vi "Channel_Manager2.vi"() -> ()   [LabVIEW 2018]
uses:
  CCDCamera/CCDCamera.lvclass
  RxTx/RxTx.lvclass
  Cooler/Cooler.lvclass
  Interface/Interface.lvclass
  Channel Manager/Channel Manager.lvclass
  Readout delay charact/Readout Delay Charact/Readout Charact.lvclass
  Save Images/Save Images.lvclass
  Product/Product.lvclass
  Creator/Creator.lvclass
panel:
  in  "Channel Manager in":refnum<class "Channel Manager.lvclass">
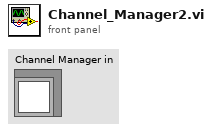
[diagram p1: front panel]
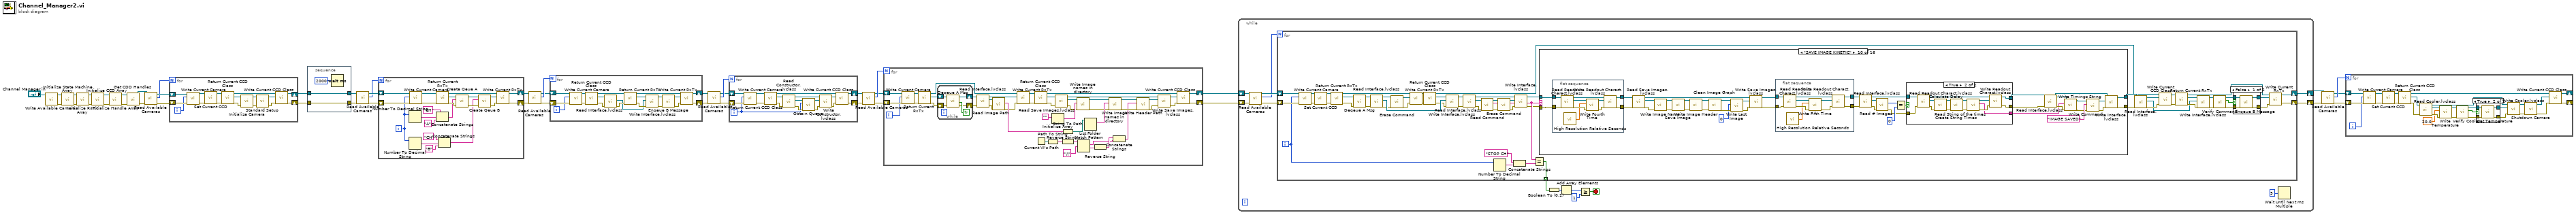
[diagram p0: block diagram]
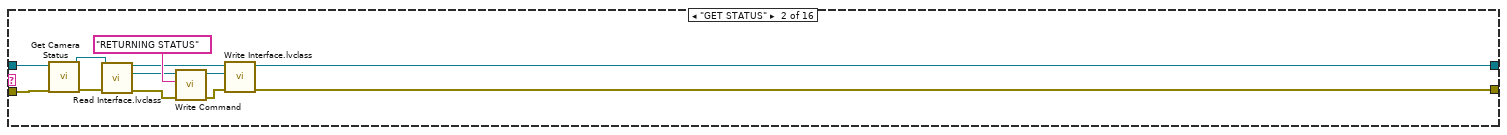
[diagram p4: hidden frame]
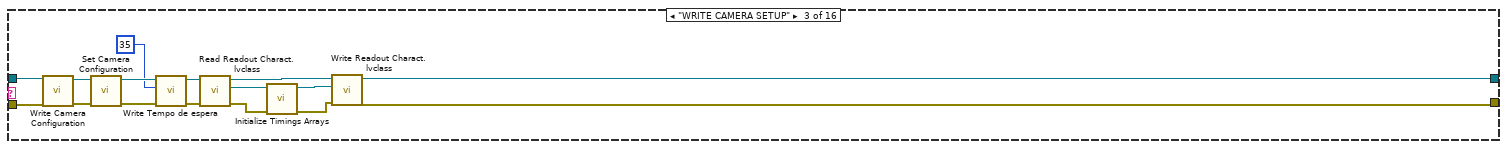
[diagram p5: hidden frame]
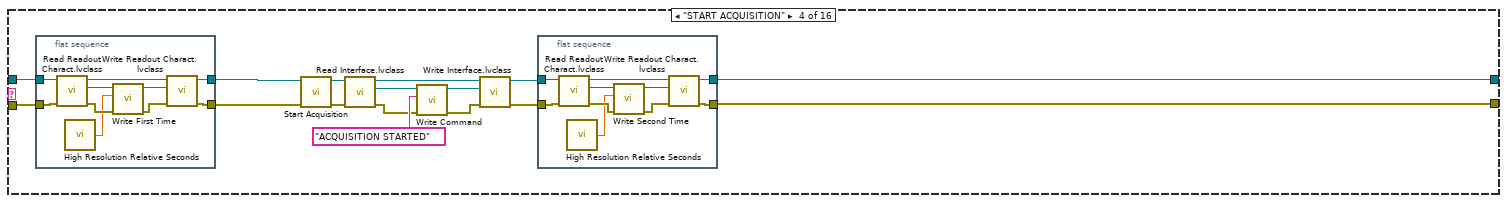
[diagram p6: hidden frame]
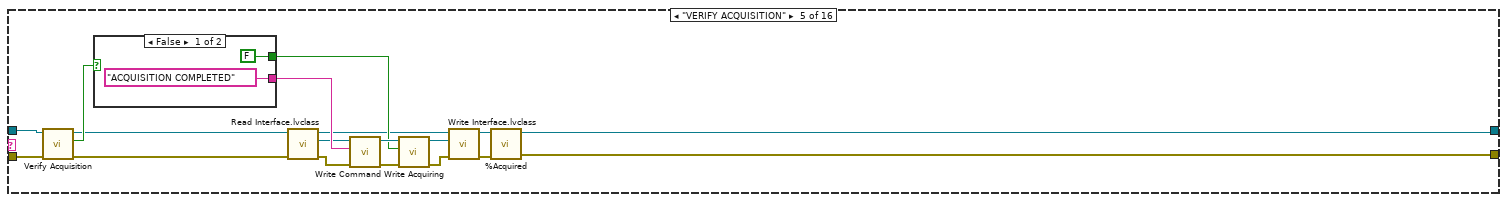
[diagram p7: hidden frame]
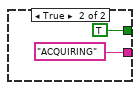
[diagram p8: hidden frame]
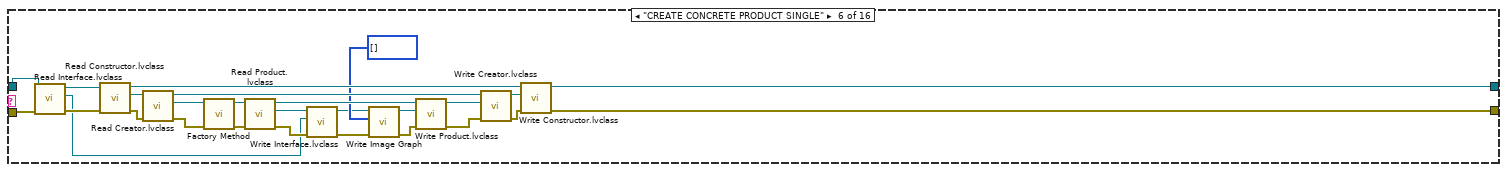
[diagram p9: hidden frame]
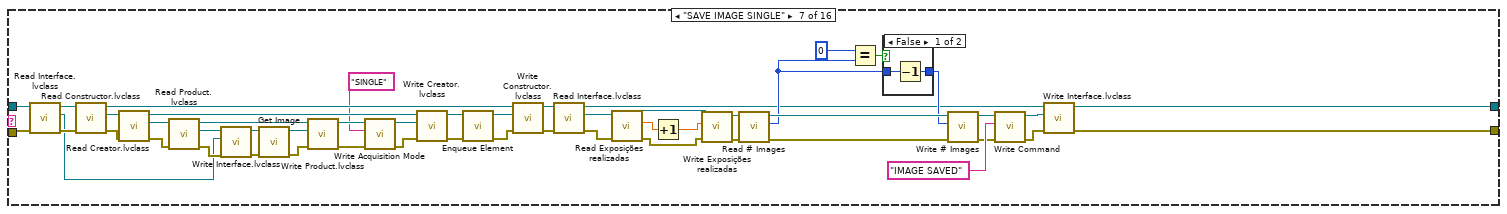
[diagram p10: hidden frame]
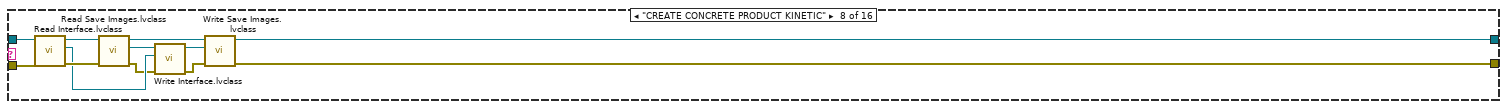
[diagram p12: hidden frame]
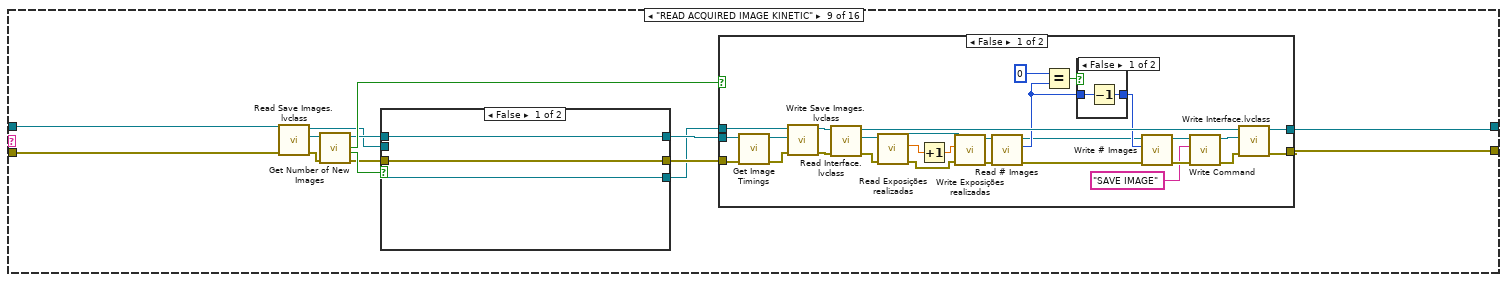
[diagram p13: hidden frame]
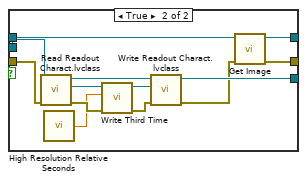
[diagram p14: hidden frame]
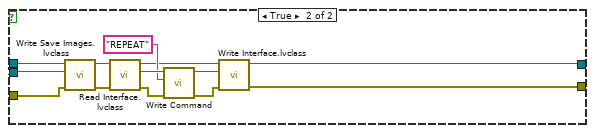
[diagram p16: hidden frame]
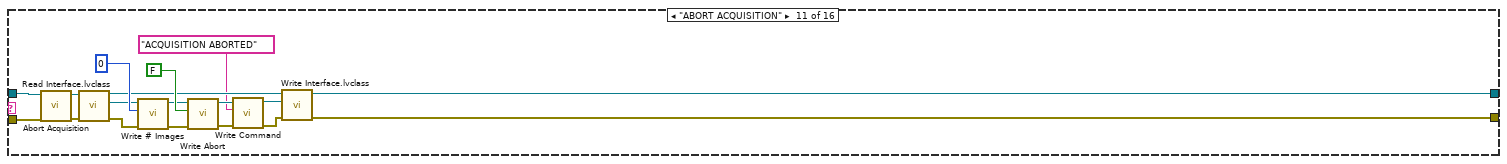
[diagram p18: hidden frame]
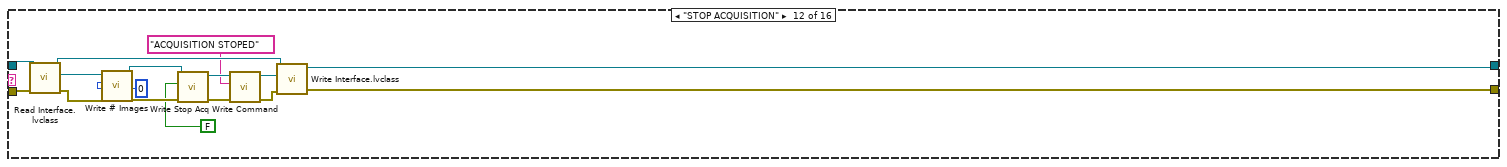
[diagram p19: hidden frame]
diagram:
  n1 = call-dynamic "Write Available Cameras.vi"("Channel Manager in"="Channel Manager in") -> ("error out"=w28:errorcluster, "Channel Manager out"=w27:refnum<class "Channel Manager.lvclass">)  [unwired: 9 in]
  n2 = call "Initialize State Machine Array.vi"("error in (no error)"=w28, "Channel Manager in"=w27) -> ("error out"=w36:errorcluster, "Channel Manager out"=w41:refnum<class "Channel Manager.lvclass">)  [unwired: 8 in]
  n3 = call "Initialize RxTx Array.vi"("error in (no error)"=w36, "Channel Manager in"=w41) -> ("error out"=w37:errorcluster, "Channel Manager out"=w40:refnum<class "Channel Manager.lvclass">)  [unwired: 8 in]
  n4 = call "Initialize CCD Array.vi"("error in (no error)"=w37, "Channel Manager in"=w40) -> ("error out"=w38:errorcluster, "Channel Manager out"=w39:refnum<class "Channel Manager.lvclass">)  [unwired: 8 in]
  n5 = call "Initialize Handle Array.vi"("error in (no error)"=w38, "Channel Manager in"=w39) -> ("error out"=w35:errorcluster, "Channel Manager out"=w34:refnum<class "Channel Manager.lvclass">)  [unwired: 8 in]
  n6 = call "Get CDD Handles.vi"("error in (no error)"=w35, "Channel Manager in"=w34) -> ("error out"=w33:errorcluster, "Channel Manager out"=w32:refnum<class "Channel Manager.lvclass">)  [unwired: 8 in]
  n7 = call-dynamic "Read Available Cameras.vi"("error in (no error)"=w33, "Channel Manager in"=w32) -> ("error out"=w30:errorcluster, "Available Cameras"=w29:u8, "Channel Manager out"=w31:refnum<class "Channel Manager.lvclass">)  [unwired: 7 in]
  n8 = for {
    N: w29 -> [_]
    shift-right: [w52] -> w45
    shift-left: w31 -> [w48]
    shift-right: [w51] -> w44
    shift-left: w30 -> [w47]
    i -> [w46]
    n9 = call-dynamic "Write Current Camera.vi"("error in (no error)"=w47, "Current Camera"=w46, "Channel Manager in"=w48) -> ("error out"=w50:errorcluster, "Channel Manager out"=w49:refnum<class "Channel Manager.lvclass">)  [unwired: 7 in]
    n10 = call "Set Current CCD.vi"("error in (no error)"=w50, "Channel Manager in"=w49) -> ("error out"=w55:errorcluster, "Channel Manager out"=w56:refnum<class "Channel Manager.lvclass">)  [unwired: 8 in]
    n11 = call "Return Current CCD Class.vi"("error in (no error)"=w55, "Channel Manager in"=w56) -> ("error out"=w60:errorcluster, "CCD Class"=w61:refnum<class "CCDCamera.lvclass">, "Channel Manager out"=w59:refnum<class "Channel Manager.lvclass">)  [unwired: 7 in]
    n12 = call "Initialize Camera.vi"("error in (no error)"=w60, "CCDCamera in"=w61) -> ("error out"=w58:errorcluster, "CCDCamera out"=w57:refnum<class "CCDCamera.lvclass">)  [unwired: 8 in]
    n13 = call "Standard Setup.vi"("error in (no error)"=w58, "CCDCamera in"=w57) -> ("error out"=w54:errorcluster, "CCDCamera out"=w53:refnum<class "CCDCamera.lvclass">)  [unwired: 8 in]
    n14 = call "Write Current CCD Class.vi"("error in (no error)"=w54, "CCD Class"=w53, "Channel Manager in"=w59) -> ("error out"=w51:errorcluster, "Channel Manager out"=w52:refnum<class "Channel Manager.lvclass">)  [unwired: 7 in]
  }
  n15 = stacked-sequence {
    tunnel: w45 -> [w63]
    tunnel: w44 -> [w62]
    tunnel: [w63] -> w24
    tunnel: [w62] -> w25
    frame #0 {
      n16 = Wait (ms)(milliseconds to wait=u32 2000) -> ()  [unwired: 1 out]
    }
  }
  n17 = call-dynamic "Read Available Cameras.vi"("error in (no error)"=w25, "Channel Manager in"=w24) -> ("error out"=w22:errorcluster, "Available Cameras"=w21:u8, "Channel Manager out"=w23:refnum<class "Channel Manager.lvclass">)  [unwired: 7 in]
  n18 = for {
    N: w21 -> [_]
    shift-right: [w71] -> w19
    shift-left: w23 -> [w66]
    shift-right: [w70] -> w20
    shift-left: w22 -> [w67]
    i -> [w65]
    n19 = Number To Decimal String(number=w65) -> (decimal integer string=w78:string)  [unwired: 1 in]
    n20 = Number To Decimal String(number=w65) -> (decimal integer string=w79:string)  [unwired: 1 in]
    n21 = call-dynamic "Write Current Camera.vi"("error in (no error)"=w67, "Current Camera"=w65, "Channel Manager in"=w66) -> ("error out"=w69:errorcluster, "Channel Manager out"=w68:refnum<class "Channel Manager.lvclass">)  [unwired: 7 in]
    n22 = call "Return Current RxTx.vi"("error in (no error)"=w69, "Channel Manager in"=w68) -> ("error out"=w86:errorcluster, "RxTx"=w76:refnum<class "RxTx.lvclass">, "Channel Manager out"=w83:refnum<class "Channel Manager.lvclass">)  [unwired: 7 in]
    n23 = Concatenate Strings("CH", w78, "A") -> (w80:string)
    n24 = Concatenate Strings("CH", w79, "B") -> (w81:string)
    n25 = call "Create Qeue A.vi"("error in (no error)"=w86, "Qeue A"=w80, "RxTx in"=w76) -> ("error out"=w84:errorcluster, "RxTx out"=w77:refnum<class "RxTx.lvclass">)  [unwired: 7 in]
    n26 = call "Create Qeue B.vi"("error in (no error)"=w84, "Qeue B"=w81, "RxTx in"=w77) -> ("error out"=w85:errorcluster, "RxTx out"=w82:refnum<class "RxTx.lvclass">)  [unwired: 7 in]
    n27 = call "Write Current RxTx.vi"("error in (no error)"=w85, "RxTx"=w82, "Channel Manager in"=w83) -> ("error out"=w70:errorcluster, "Channel Manager out"=w71:refnum<class "Channel Manager.lvclass">)  [unwired: 7 in]
  }
  n28 = call-dynamic "Read Available Cameras.vi"("error in (no error)"=w20, "Channel Manager in"=w19) -> ("error out"=w16:errorcluster, "Available Cameras"=w18:u8, "Channel Manager out"=w17:refnum<class "Channel Manager.lvclass">)  [unwired: 7 in]
  n29 = for {
    N: w18 -> [_]
    shift-right: [w93] -> w14
    shift-left: w17 -> [w89]
    shift-right: [w92] -> w15
    shift-left: w16 -> [w88]
    i -> [w87]
    n30 = call-dynamic "Write Current Camera.vi"("error in (no error)"=w88, "Current Camera"=w87, "Channel Manager in"=w89) -> ("error out"=w91:errorcluster, "Channel Manager out"=w90:refnum<class "Channel Manager.lvclass">)  [unwired: 7 in]
    n31 = call "Return Current CCD Class.vi"("error in (no error)"=w91, "Channel Manager in"=w90) -> ("error out"=w104:errorcluster, "CCD Class"=w105:refnum<class "CCDCamera.lvclass">, "Channel Manager out"=w102:refnum<class "Channel Manager.lvclass">)  [unwired: 7 in]
    n32 = call-dynamic "Read Interface.lvclass.vi"("error in (no error)"=w104, "CCDCamera in"=w105) -> ("error out"=w103:errorcluster, "Interface.lvclass"=w99:refnum<class "Interface.lvclass">)  [unwired: 7 in, 1 out]
    n33 = call "Return Current RxTx.vi"("error in (no error)"=w103, "Channel Manager in"=w102) -> ("error out"=w101:errorcluster, "RxTx"=w100:refnum<class "RxTx.lvclass">, "Channel Manager out"=w96:refnum<class "Channel Manager.lvclass">)  [unwired: 7 in]
    n34 = call-dynamic "Write Interface.lvclass.vi"("error in (no error)"=w101, "Interface.lvclass"=w99, "RxTx in"=w100) -> ("error out"=w98:errorcluster, "RxTx out"=w97:refnum<class "RxTx.lvclass">)  [unwired: 7 in]
    n35 = call "Enqeue B Message.vi"("error in (no error)"=w98, "RxTx in"=w97) -> ("error out"=w94:errorcluster, "RxTx out"=w95:refnum<class "RxTx.lvclass">)  [unwired: 8 in]
    n36 = call "Write Current RxTx.vi"("error in (no error)"=w94, "RxTx"=w95, "Channel Manager in"=w96) -> ("error out"=w92:errorcluster, "Channel Manager out"=w93:refnum<class "Channel Manager.lvclass">)  [unwired: 7 in]
  }
  n37 = call-dynamic "Read Available Cameras.vi"("error in (no error)"=w15, "Channel Manager in"=w14) -> ("error out"=w11:errorcluster, "Available Cameras"=w13:u8, "Channel Manager out"=w12:refnum<class "Channel Manager.lvclass">)  [unwired: 7 in]
  n38 = for {
    N: w13 -> [_]
    shift-right: [w112] -> w9
    shift-left: w12 -> [w108]
    shift-right: [w111] -> w10
    shift-left: w11 -> [w107]
    i -> [w106]
    n39 = call-dynamic "Write Current Camera.vi"("error in (no error)"=w107, "Current Camera"=w106, "Channel Manager in"=w108) -> ("error out"=w110:errorcluster, "Channel Manager out"=w109:refnum<class "Channel Manager.lvclass">)  [unwired: 7 in]
    n40 = call "Return Current CCD Class.vi"("error in (no error)"=w110, "Channel Manager in"=w109) -> ("error out"=w121:errorcluster, "CCD Class"=w122:refnum<class "CCDCamera.lvclass">, "Channel Manager out"=w113:refnum<class "Channel Manager.lvclass">)  [unwired: 7 in]
    n41 = call "Read Constructor.lvclass.vi"("error in (no error)"=w121, "CCDCamera in"=w122) -> ("error out"=w119:errorcluster, "Constructor.lvclass"=w120:refnum<class "Constructor.lvclass">, "CCDCamera out"=w116:refnum<class "CCDCamera.lvclass">)  [unwired: 7 in]
    n42 = call "Obtain Queue.vi"("error in (no error)"=w119, "Channel"=w106, "Constructor in"=w120) -> ("error out"=w118:errorcluster, "Constructor out"=w117:refnum<class "Constructor.lvclass">)  [unwired: 7 in]
    n43 = call "Write Constructor.lvclass.vi"("error in (no error)"=w118, "Constructor.lvclass"=w117, "CCDCamera in"=w116) -> ("error out"=w115:errorcluster, "CCDCamera out"=w114:refnum<class "CCDCamera.lvclass">)  [unwired: 7 in]
    n44 = call "Write Current CCD Class.vi"("error in (no error)"=w115, "CCD Class"=w114, "Channel Manager in"=w113) -> ("error out"=w111:errorcluster, "Channel Manager out"=w112:refnum<class "Channel Manager.lvclass">)  [unwired: 7 in]
  }
  n45 = call-dynamic "Read Available Cameras.vi"("error in (no error)"=w10, "Channel Manager in"=w9) -> ("error out"=w6:errorcluster, "Available Cameras"=w8:u8, "Channel Manager out"=w7:refnum<class "Channel Manager.lvclass">)  [unwired: 7 in]
  n46 = for {
    N: w8 -> [_]
    shift-right: [w159] -> w42
    shift-left: w7 -> [w154]
    shift-right: [w158] -> w43
    shift-left: w6 -> [w155]
    i -> [w153]
    n47 = call-dynamic "Write Current Camera.vi"("error in (no error)"=w155, "Current Camera"=w153, "Channel Manager in"=w154) -> ("error out"=w157:errorcluster, "Channel Manager out"=w156:refnum<class "Channel Manager.lvclass">)  [unwired: 7 in]
    n48 = call "Return Current RxTx.vi"("error in (no error)"=w157, "Channel Manager in"=w156) -> ("error out"=w167:errorcluster, "RxTx"=w166:refnum<class "RxTx.lvclass">, "Channel Manager out"=w162:refnum<class "Channel Manager.lvclass">)  [unwired: 7 in]
    n49 = while {
      shift-right: [w170] -> w164
      shift-left: w166 -> [w169]
      shift-right: [w171] -> w165
      shift-left: w167 -> [w168]
      stop <- w172 continue-if-true
      n50 = call "Deqeue A Msg.vi"("error in (no error)"=w168, "RxTx in"=w169) -> ("error out"=w171:errorcluster, "Timeout"=w172:bool, "RxTx out"=w170:refnum<class "RxTx.lvclass">)  [unwired: 7 in]
    }
    n51 = call-dynamic "Read Interface.lvclass.vi"("error in (no error)"=w165, "RxTx in"=w164) -> ("error out"=w141:errorcluster, "Interface.lvclass"=w142:refnum<class "Interface.lvclass">, "RxTx out"=w163:refnum<class "RxTx.lvclass">)  [unwired: 7 in]
    n52 = call-dynamic "Read Image Path.vi"("error in (no error)"=w141, "Interface in"=w142) -> ("error out"=w135:errorcluster, "Image Path"=w152:string)  [unwired: 7 in, 1 out]
    n53 = call "Write Current RxTx.vi"("error in (no error)"=w135, "RxTx"=w163, "Channel Manager in"=w162) -> ("error out"=w160:errorcluster, "Channel Manager out"=w161:refnum<class "Channel Manager.lvclass">)  [unwired: 7 in]
    n54 = call "Return Current CCD Class.vi"("error in (no error)"=w160, "Channel Manager in"=w161) -> ("error out"=w139:errorcluster, "CCD Class"=w140:refnum<class "CCDCamera.lvclass">, "Channel Manager out"=w136:refnum<class "Channel Manager.lvclass">)  [unwired: 7 in]
    n55 = Current VI's Path() -> (path=w130:path)
    n56 = Path To String(path=w130) -> (string=w129:string)
    n57 = Initialize Array("") -> (w147:string[])  [unwired: 1 in]
    n58 = call "Read Save Images.lvclass.vi"("error in (no error)"=w139, "CCDCamera in"=w140) -> ("error out"=w146:errorcluster, "Save Images.lvclass"=w145:refnum<class "Save Images.lvclass">, "CCDCamera out"=w144:refnum<class "CCDCamera.lvclass">)  [unwired: 7 in]
    n59 = Reverse String(1:w129) -> (0:w128:string)
    n60 = String To Path(string=w152) -> (path=w151:path)
    n61 = call "Write Image names in directory.vi"("error in (no error)"=w146, "Image names in directory"=w147, "Save Images in"=w145) -> ("error out"=w149:errorcluster, "Save Images out"=w148:refnum<class "Save Images.lvclass">)  [unwired: 7 in]
    n62 = Match Pattern(string=w128, regular expression="\\") -> (match substring=w124:string, after substring=w126:string)  [unwired: 1 in, 2 out]
    n63 = List Folder(path=w151) -> (filenames=w150:string[])  [unwired: 3 in, 3 out]
    n64 = Reverse String(1:w126) -> (0:w125:string)
    n65 = call "Write Image names in directory.vi"("error in (no error)"=w149, "Image names in directory"=w150, "Save Images in"=w148) -> ("error out"=w132:errorcluster, "Save Images out"=w133:refnum<class "Save Images.lvclass">)  [unwired: 7 in]
    n66 = Concatenate Strings(w125, w124) -> (w123:string)
    n67 = call-dynamic "Write Header Path.vi"("error in (no error)"=w132, "Header Path"=w123, "Save Images in"=w133) -> ("error out"=w131:errorcluster, "Save Images out"=w134:refnum<class "Save Images.lvclass">)  [unwired: 7 in]
    n68 = call "Write Save Images.lvclass.vi"("error in (no error)"=w131, "Save Images.lvclass"=w134, "CCDCamera in"=w144) -> ("error out"=w137:errorcluster, "CCDCamera out"=w138:refnum<class "CCDCamera.lvclass">)  [unwired: 7 in]
    n69 = call "Write Current CCD Class.vi"("error in (no error)"=w137, "CCD Class"=w138, "Channel Manager in"=w136) -> ("error out"=w158:errorcluster, "Channel Manager out"=w159:refnum<class "Channel Manager.lvclass">)  [unwired: 7 in]
  }
  n70 = while {
    shift-right: [w179] -> w4
    shift-left: w42 -> [w176]
    shift-right: [w178] -> w5
    shift-left: w43 -> [w177]
    stop <- w181 stop-if-true
    n71 = call-dynamic "Read Available Cameras.vi"("error in (no error)"=w177, "Channel Manager in"=w176) -> ("error out"=w174:errorcluster, "Available Cameras"=w173:u8, "Channel Manager out"=w175:refnum<class "Channel Manager.lvclass">)  [unwired: 7 in]
    n72 = for {
      N: w173 -> [_]
      tunnel: [w209] -> w185 mode=indexing
      shift-right: [w192] -> w179
      shift-left: w175 -> [w188]
      shift-right: [w191] -> w178
      shift-left: w174 -> [w187]
      i -> [w186]
      n73 = call-dynamic "Write Current Camera.vi"("error in (no error)"=w187, "Current Camera"=w186, "Channel Manager in"=w188) -> ("error out"=w190:errorcluster, "Channel Manager out"=w189:refnum<class "Channel Manager.lvclass">)  [unwired: 7 in]
      n74 = call "Set Current CCD.vi"("error in (no error)"=w190, "Channel Manager in"=w189) -> ("error out"=w235:errorcluster, "Channel Manager out"=w236:refnum<class "Channel Manager.lvclass">)  [unwired: 8 in]
      n75 = call "Return Current RxTx.vi"("error in (no error)"=w235, "Channel Manager in"=w236) -> ("error out"=w208:errorcluster, "RxTx"=w207:refnum<class "RxTx.lvclass">, "Channel Manager out"=w239:refnum<class "Channel Manager.lvclass">)  [unwired: 7 in]
      n76 = call "Deqeue A Msg.vi"("error in (no error)"=w208, "RxTx in"=w207) -> ("error out"=w198:errorcluster, "RxTx out"=w197:refnum<class "RxTx.lvclass">)  [unwired: 7 in, 1 out]
      n77 = call-dynamic "Read Interface.lvclass.vi"("error in (no error)"=w198, "RxTx in"=w197) -> ("error out"=w196:errorcluster, "Interface.lvclass"=w241:refnum<class "Interface.lvclass">, "RxTx out"=w195:refnum<class "RxTx.lvclass">)  [unwired: 7 in]
      n78 = call "Erase Command.vi"("error in (no error)"=w196, "RxTx in"=w195) -> ("error out"=w193:errorcluster, "RxTx out"=w194:refnum<class "RxTx.lvclass">)  [unwired: 8 in]
      n79 = call "Write Current RxTx.vi"("error in (no error)"=w193, "RxTx"=w194, "Channel Manager in"=w239) -> ("error out"=w238:errorcluster, "Channel Manager out"=w237:refnum<class "Channel Manager.lvclass">)  [unwired: 7 in]
      n80 = call "Return Current CCD Class.vi"("error in (no error)"=w238, "Channel Manager in"=w237) -> ("error out"=w240:errorcluster, "CCD Class"=w242:refnum<class "CCDCamera.lvclass">, "Channel Manager out"=w222:refnum<class "Channel Manager.lvclass">)  [unwired: 7 in]
      n81 = call-dynamic "Write Interface.lvclass.vi"("error in (no error)"=w240, "Interface.lvclass"=w241, "CCDCamera in"=w242) -> ("error out"=w228:errorcluster, "CCDCamera out"=w229:refnum<class "CCDCamera.lvclass">)  [unwired: 7 in]
      n82 = call-dynamic "Read Interface.lvclass.vi"("error in (no error)"=w228, "CCDCamera in"=w229) -> ("error out"=w233:errorcluster, "Interface.lvclass"=w234:refnum<class "Interface.lvclass">, "CCDCamera out"=w206:refnum<class "CCDCamera.lvclass">)  [unwired: 7 in]
      n83 = call "Read Command.vi"("error in (no error)"=w233, "Interface in"=w234) -> ("error out"=w202:errorcluster, "Command"=w232:string, "Interface out"=w201:refnum<class "Interface.lvclass">)  [unwired: 7 in]
      n84 = Number To Decimal String(number=w186) -> (decimal integer string=w226:string)  [unwired: 1 in]
      n85 = call "Erase Command.vi"("error in (no error)"=w202, "Interface in"=w201) -> ("error out"=w199:errorcluster, "Interface out"=w200:refnum<class "Interface.lvclass">)  [unwired: 8 in]
      n86 = Concatenate Strings("STOP CH", w226) -> (w225:string)
      n87 = call-dynamic "Write Interface.lvclass.vi"("error in (no error)"=w199, "Interface.lvclass"=w200, "CCDCamera in"=w206) -> ("error out"=w204:errorcluster, "CCDCamera out"=w205:refnum<class "CCDCamera.lvclass">)  [unwired: 7 in]
      n88 = Equal?(x=w232, y=w225) -> (x = y?=w209:bool)
      n89 = case shown="\"SAVE IMAGE KINETIC\"" w232 {
        tunnel: w205 -> [w250 w262 w277 w285 w332 w347 w394 w428 w435 w525 w599 w612 w618 w630 w642 w655]
        tunnel: w204 -> [w249 w261 w278 w286 w331 w348 w395 w427 w434 w524 w600 w611 w617 w629 w641 w654]
        tunnel: [w250 w252 w264 w280 w318 w355 w410 w429 w431 w542 w588 w607 w618 w631 w639 w653] -> w230
        tunnel: [w249 w251 w263 w279 w317 w354 w409 w418 w430 w543 w589 w606 w617 w632 w640 w652] -> w231
        frame "False", Default {
        }
        frame "GET STATUS" {
          n90 = call "Get Camera Status.vi"("error in (no error)"=w261, "CCDCamera in"=w262) -> ("error out"=w260:errorcluster, "CCDCamera out"=w259:refnum<class "CCDCamera.lvclass">)  [unwired: 7 in, 1 out]
          n91 = call-dynamic "Read Interface.lvclass.vi"("error in (no error)"=w260, "CCDCamera in"=w259) -> ("error out"=w256:errorcluster, "Interface.lvclass"=w257:refnum<class "Interface.lvclass">, "CCDCamera out"=w253:refnum<class "CCDCamera.lvclass">)  [unwired: 7 in]
          n92 = call "Write Command.vi"("error in (no error)"=w256, "Command"="RETURNING STATUS", "Interface in"=w257) -> ("error out"=w255:errorcluster, "Interface out"=w254:refnum<class "Interface.lvclass">)  [unwired: 7 in]
          n93 = call-dynamic "Write Interface.lvclass.vi"("error in (no error)"=w255, "Interface.lvclass"=w254, "CCDCamera in"=w253) -> ("error out"=w251:errorcluster, "CCDCamera out"=w252:refnum<class "CCDCamera.lvclass">)  [unwired: 7 in]
        }
        frame "WRITE CAMERA SETUP" {
          n94 = call-dynamic "Write Camera Configuration.vi"("error in (no error)"=w278, "CCDCamera in"=w277) -> ("error out"=w276:errorcluster, "CCDCamera out"=w275:refnum<class "CCDCamera.lvclass">)  [unwired: 8 in]
          n95 = call "Set Camera Configuration.vi"("error in (no error)"=w276, "CCDCamera in"=w275) -> ("error out"=w274:errorcluster, "CCDCamera out"=w273:refnum<class "CCDCamera.lvclass">)  [unwired: 8 in]
          n96 = call-dynamic "Write Tempo de espera.vi"("error in (no error)"=w274, "Tempo de espera"=u16 35, "CCDCamera in"=w273) -> ("error out"=w271:errorcluster, "CCDCamera out"=w270:refnum<class "CCDCamera.lvclass">)  [unwired: 7 in]
          n97 = call-dynamic "Read Readout Charact.lvclass.vi"("error in (no error)"=w271, "CCDCamera in"=w270) -> ("error out"=w266:errorcluster, "Readout Charact.lvclass"=w269:refnum<class "Readout Charact.lvclass">, "CCDCamera out"=w265:refnum<class "CCDCamera.lvclass">)  [unwired: 7 in]
          n98 = call "Initialize Timings Arrays.vi"("error in (no error)"=w266, "Readout Charact in"=w269) -> ("error out"=w267:errorcluster, "Readout Charact out"=w268:refnum<class "Readout Charact.lvclass">)  [unwired: 8 in]
          n99 = call-dynamic "Write Readout Charact.lvclass.vi"("error in (no error)"=w267, "Readout Charact.lvclass"=w268, "CCDCamera in"=w265) -> ("error out"=w263:errorcluster, "CCDCamera out"=w264:refnum<class "CCDCamera.lvclass">)  [unwired: 7 in]
        }
        frame "START ACQUISITION" {
          n100 = flat-sequence {
            tunnel: w286 -> [w314]
            tunnel: w285 -> [w313]
            tunnel: [w312] -> w284
            tunnel: [w311] -> w283
            frame #0 {
              n101 = call-dynamic "Read Readout Charact.lvclass.vi"("error in (no error)"=w314, "CCDCamera in"=w313) -> ("error out"=w308:errorcluster, "Readout Charact.lvclass"=w309:refnum<class "Readout Charact.lvclass">, "CCDCamera out"=w305:refnum<class "CCDCamera.lvclass">)  [unwired: 7 in]
              n102 = call <vilib>:"High Resolution Relative Seconds.vi"() -> ("relative seconds"=w306:dbl)
              n103 = call-dynamic "Write First Time.vi"("error in (no error)"=w308, "First Time"=w306, "Readout Charact in"=w309) -> ("error out"=w307:errorcluster, "Readout Charact out"=w310:refnum<class "Readout Charact.lvclass">)  [unwired: 7 in]
              n104 = call-dynamic "Write Readout Charact.lvclass.vi"("error in (no error)"=w307, "Readout Charact.lvclass"=w310, "CCDCamera in"=w305) -> ("error out"=w311:errorcluster, "CCDCamera out"=w312:refnum<class "CCDCamera.lvclass">)  [unwired: 7 in]
            }
          }
          n105 = call "Start Acquisition.vi"("error in (no error)"=w283, "CCDCamera in"=w284) -> ("error out"=w292:errorcluster, "CCDCamera out"=w293:refnum<class "CCDCamera.lvclass">)  [unwired: 8 in]
          n106 = call-dynamic "Read Interface.lvclass.vi"("error in (no error)"=w292, "CCDCamera in"=w293) -> ("error out"=w287:errorcluster, "Interface.lvclass"=w291:refnum<class "Interface.lvclass">, "CCDCamera out"=w289:refnum<class "CCDCamera.lvclass">)  [unwired: 7 in]
          n107 = call "Write Command.vi"("error in (no error)"=w287, "Command"="ACQUISITION STARTED", "Interface in"=w291) -> ("error out"=w288:errorcluster, "Interface out"=w290:refnum<class "Interface.lvclass">)  [unwired: 7 in]
          n108 = call-dynamic "Write Interface.lvclass.vi"("error in (no error)"=w288, "Interface.lvclass"=w290, "CCDCamera in"=w289) -> ("error out"=w281:errorcluster, "CCDCamera out"=w282:refnum<class "CCDCamera.lvclass">)  [unwired: 7 in]
          n109 = flat-sequence {
            tunnel: w281 -> [w304]
            tunnel: w282 -> [w303]
            tunnel: [w302] -> w280
            tunnel: [w301] -> w279
            frame #0 {
              n110 = call-dynamic "Read Readout Charact.lvclass.vi"("error in (no error)"=w304, "CCDCamera in"=w303) -> ("error out"=w296:errorcluster, "Readout Charact.lvclass"=w297:refnum<class "Readout Charact.lvclass">, "CCDCamera out"=w300:refnum<class "CCDCamera.lvclass">)  [unwired: 7 in]
              n111 = call <vilib>:"High Resolution Relative Seconds.vi"() -> ("relative seconds"=w295:dbl)
              n112 = call-dynamic "Write Second Time.vi"("error in (no error)"=w296, "Second Time"=w295, "Readout Charact in"=w297) -> ("error out"=w299:errorcluster, "Readout Charact out"=w298:refnum<class "Readout Charact.lvclass">)  [unwired: 7 in]
              n113 = call-dynamic "Write Readout Charact.lvclass.vi"("error in (no error)"=w299, "Readout Charact.lvclass"=w298, "CCDCamera in"=w300) -> ("error out"=w301:errorcluster, "CCDCamera out"=w302:refnum<class "CCDCamera.lvclass">)  [unwired: 7 in]
            }
          }
        }
        frame "VERIFY ACQUISITION" {
          n114 = call "Verify Acquisition.vi"("error in (no error)"=w331, "CCDCamera in"=w332) -> ("error out"=w315:errorcluster, "Acquiring"=w330:bool, "CCDCamera out"=w316:refnum<class "CCDCamera.lvclass">)  [unwired: 7 in]
          n115 = case shown="False" w330 {
            tunnel: ["ACQUISITION COMPLETED" "ACQUIRING"] -> w329
            tunnel: [FALSE ("Acquiring") TRUE ("Acquiring")] -> w326
            frame False {
            }
            frame True {
            }
          }
          n116 = call-dynamic "Read Interface.lvclass.vi"("error in (no error)"=w315, "CCDCamera in"=w316) -> ("error out"=w324:errorcluster, "Interface.lvclass"=w325:refnum<class "Interface.lvclass">, "CCDCamera out"=w321:refnum<class "CCDCamera.lvclass">)  [unwired: 7 in]
          n117 = call "Write Command.vi"("error in (no error)"=w324, "Command"=w329, "Interface in"=w325) -> ("error out"=w328:errorcluster, "Interface out"=w327:refnum<class "Interface.lvclass">)  [unwired: 7 in]
          n118 = call-dynamic "Write Acquiring.vi"("error in (no error)"=w328, "Acquiring"=w326, "Interface in"=w327) -> ("error out"=w323:errorcluster, "Interface out"=w322:refnum<class "Interface.lvclass">)  [unwired: 7 in]
          n119 = call-dynamic "Write Interface.lvclass.vi"("error in (no error)"=w323, "Interface.lvclass"=w322, "CCDCamera in"=w321) -> ("error out"=w320:errorcluster, "CCDCamera out"=w319:refnum<class "CCDCamera.lvclass">)  [unwired: 7 in]
          n120 = call "%Acquired.vi"("error in (no error)"=w320, "CCDCamera in"=w319) -> ("error out"=w317:errorcluster, "CCDCamera out"=w318:refnum<class "CCDCamera.lvclass">)  [unwired: 8 in]
        }
        frame "CREATE CONCRETE PRODUCT SINGLE" {
          n121 = call-dynamic "Read Interface.lvclass.vi"("error in (no error)"=w348, "CCDCamera in"=w347) -> ("error out"=w345:errorcluster, "Interface.lvclass"=w342:refnum<class "Interface.lvclass">, "CCDCamera out"=w346:refnum<class "CCDCamera.lvclass">)  [unwired: 7 in]
          n122 = call "Read Constructor.lvclass.vi"("error in (no error)"=w345, "CCDCamera in"=w346) -> ("error out"=w358:errorcluster, "Constructor.lvclass"=w359:refnum<class "Constructor.lvclass">, "CCDCamera out"=w363:refnum<class "CCDCamera.lvclass">)  [unwired: 7 in]
          n123 = call "Read Creator.lvclass.vi"("error in (no error)"=w358, "Constructor in"=w359) -> ("error out"=w357:errorcluster, "Creator.lvclass"=w356:refnum<class "Creator.lvclass">, "Constructor out"=w362:refnum<class "Constructor.lvclass">)  [unwired: 7 in]
          n124 = call-dynamic "Factory Method.vi"("error in (no error)"=w357, "Creator in"=w356) -> ("error out"=w353:errorcluster, "Creator out"=w352:refnum<class "Creator.lvclass">)  [unwired: 8 in]
          n125 = call "Read Product.lvclass.vi"("error in (no error)"=w353, "Creator in"=w352) -> ("error out"=w344:errorcluster, "Product.lvclass"=w343:refnum<class "Product.lvclass">, "Creator out"=w351:refnum<class "Creator.lvclass">)  [unwired: 7 in]
          n126 = call "Write Interface.lvclass.vi"("error in (no error)"=w344, "Interface.lvclass"=w342, "Product in"=w343) -> ("error out"=w340:errorcluster, "Product out"=w339:refnum<class "Product.lvclass">)  [unwired: 7 in]
          n127 = call "Write Image Graph.vi"("error in (no error)"=w340, "Image Graph"=u16[] [], "Product in"=w339) -> ("error out"=w337:errorcluster, "Product out"=w338:refnum<class "Product.lvclass">)  [unwired: 7 in]
          n128 = call "Write Product.lvclass.vi"("error in (no error)"=w337, "Product.lvclass"=w338, "Creator in"=w351) -> ("error out"=w350:errorcluster, "Creator out"=w349:refnum<class "Creator.lvclass">)  [unwired: 7 in]
          n129 = call "Write Creator.lvclass.vi"("error in (no error)"=w350, "Creator.lvclass"=w349, "Constructor in"=w362) -> ("error out"=w361:errorcluster, "Constructor out"=w360:refnum<class "Constructor.lvclass">)  [unwired: 7 in]
          n130 = call "Write Constructor.lvclass.vi"("error in (no error)"=w361, "Constructor.lvclass"=w360, "CCDCamera in"=w363) -> ("error out"=w354:errorcluster, "CCDCamera out"=w355:refnum<class "CCDCamera.lvclass">)  [unwired: 7 in]
        }
        frame "SAVE IMAGE SINGLE" {
          n131 = call-dynamic "Read Interface.lvclass.vi"("error in (no error)"=w395, "CCDCamera in"=w394) -> ("error out"=w392:errorcluster, "Interface.lvclass"=w385:refnum<class "Interface.lvclass">, "CCDCamera out"=w393:refnum<class "CCDCamera.lvclass">)  [unwired: 7 in]
          n132 = call "Read Constructor.lvclass.vi"("error in (no error)"=w392, "CCDCamera in"=w393) -> ("error out"=w390:errorcluster, "Constructor.lvclass"=w391:refnum<class "Constructor.lvclass">, "CCDCamera out"=w378:refnum<class "CCDCamera.lvclass">)  [unwired: 7 in]
          n133 = call "Read Creator.lvclass.vi"("error in (no error)"=w390, "Constructor in"=w391) -> ("error out"=w388:errorcluster, "Creator.lvclass"=w389:refnum<class "Creator.lvclass">, "Constructor out"=w379:refnum<class "Constructor.lvclass">)  [unwired: 7 in]
          n134 = call "Read Product.lvclass.vi"("error in (no error)"=w388, "Creator in"=w389) -> ("error out"=w386:errorcluster, "Product.lvclass"=w387:refnum<class "Product.lvclass">, "Creator out"=w380:refnum<class "Creator.lvclass">)  [unwired: 7 in]
          n135 = call "Write Interface.lvclass.vi"("error in (no error)"=w386, "Interface.lvclass"=w385, "Product in"=w387) -> ("error out"=w383:errorcluster, "Product out"=w384:refnum<class "Product.lvclass">)  [unwired: 7 in]
          n136 = call-dynamic "Get Image.vi"("error in (no error)"=w383, "Product in"=w384) -> ("error out"=w382:errorcluster, "Product out"=w381:refnum<class "Product.lvclass">)  [unwired: 8 in]
          n137 = call "Write Product.lvclass.vi"("error in (no error)"=w382, "Product.lvclass"=w381, "Creator in"=w380) -> ("error out"=w365:errorcluster, "Creator out"=w366:refnum<class "Creator.lvclass">)  [unwired: 7 in]
          n138 = call "Write Acquisition Mode.vi"("error in (no error)"=w365, "Acquisition Mode"="SINGLE", "Creator in"=w366) -> ("error out"=w368:errorcluster, "Creator out"=w367:refnum<class "Creator.lvclass">)  [unwired: 7 in]
          n139 = call "Write Creator.lvclass.vi"("error in (no error)"=w368, "Creator.lvclass"=w367, "Constructor in"=w379) -> ("error out"=w372:errorcluster, "Constructor out"=w371:refnum<class "Constructor.lvclass">)  [unwired: 7 in]
          n140 = call "Enqueue Element.vi"("error in (no error)"=w372, "Constructor in"=w371) -> ("error out"=w369:errorcluster, "Constructor out"=w370:refnum<class "Constructor.lvclass">)  [unwired: 8 in]
          n141 = call "Write Constructor.lvclass.vi"("error in (no error)"=w369, "Constructor.lvclass"=w370, "CCDCamera in"=w378) -> ("error out"=w377:errorcluster, "CCDCamera out"=w376:refnum<class "CCDCamera.lvclass">)  [unwired: 7 in]
          n142 = call-dynamic "Read Interface.lvclass.vi"("error in (no error)"=w377, "CCDCamera in"=w376) -> ("error out"=w374:errorcluster, "Interface.lvclass"=w375:refnum<class "Interface.lvclass">, "CCDCamera out"=w373:refnum<class "CCDCamera.lvclass">)  [unwired: 7 in]
          n143 = call-dynamic "Read Exposições realizadas.vi"("error in (no error)"=w374, "Interface in"=w375) -> ("error out"=w411:errorcluster, "Exposições realizadas"=w414:dbl, "Interface out"=w412:refnum<class "Interface.lvclass">)  [unwired: 7 in]
          n144 = Increment(x=w414) -> (x+1=w413:dbl)
          n145 = call-dynamic "Write Exposições realizadas.vi"("error in (no error)"=w411, "Exposições realizadas"=w413, "Interface in"=w412) -> ("error out"=w405:errorcluster, "Interface out"=w404:refnum<class "Interface.lvclass">)  [unwired: 7 in]
          n146 = call-dynamic "Read # Images.vi"("error in (no error)"=w405, "Interface in"=w404) -> ("error out"=w402:errorcluster, "# Images"=w396:u32, "Interface out"=w403:refnum<class "Interface.lvclass">)  [unwired: 7 in]
          n147 = Equal?(x=u32 0, y=w396) -> (x = y?=w399:bool)
          n148 = case shown="False" w399 {
            tunnel: [w416 w417] -> w397
            tunnel: w396 -> [w415 w417]
            frame False {
              n149 = Decrement(x=w415) -> (x-1=w416:u32)
            }
            frame True {
            }
          }
          n150 = call-dynamic "Write # Images.vi"("error in (no error)"=w402, "# Images"=w397, "Interface in"=w403) -> ("error out"=w401:errorcluster, "Interface out"=w400:refnum<class "Interface.lvclass">)  [unwired: 7 in]
          n151 = call "Write Command.vi"("error in (no error)"=w401, "Command"="IMAGE SAVED", "Interface in"=w400) -> ("error out"=w408:errorcluster, "Interface out"=w407:refnum<class "Interface.lvclass">)  [unwired: 7 in]
          n152 = call-dynamic "Write Interface.lvclass.vi"("error in (no error)"=w408, "Interface.lvclass"=w407, "CCDCamera in"=w373) -> ("error out"=w409:errorcluster, "CCDCamera out"=w410:refnum<class "CCDCamera.lvclass">)  [unwired: 7 in]
        }
        frame "CREATE CONCRETE PRODUCT KINETIC" {
          n153 = call-dynamic "Read Interface.lvclass.vi"("error in (no error)"=w427, "CCDCamera in"=w428) -> ("error out"=w425:errorcluster, "Interface.lvclass"=w424:refnum<class "Interface.lvclass">, "CCDCamera out"=w426:refnum<class "CCDCamera.lvclass">)  [unwired: 7 in]
          n154 = call "Read Save Images.lvclass.vi"("error in (no error)"=w425, "CCDCamera in"=w426) -> ("error out"=w422:errorcluster, "Save Images.lvclass"=w423:refnum<class "Save Images.lvclass">, "CCDCamera out"=w419:refnum<class "CCDCamera.lvclass">)  [unwired: 7 in]
          n155 = call-dynamic "Write Interface.lvclass.vi"("error in (no error)"=w422, "Interface.lvclass"=w424, "Save Images in"=w423) -> ("error out"=w421:errorcluster, "Save Images out"=w420:refnum<class "Save Images.lvclass">)  [unwired: 7 in]
          n156 = call "Write Save Images.lvclass.vi"("error in (no error)"=w421, "Save Images.lvclass"=w420, "CCDCamera in"=w419) -> ("error out"=w418:errorcluster, "CCDCamera out"=w429:refnum<class "CCDCamera.lvclass">)  [unwired: 7 in]
        }
        frame "READ ACQUIRED IMAGE KINETIC" {
          n157 = call "Read Save Images.lvclass.vi"("error in (no error)"=w434, "CCDCamera in"=w435) -> ("error out"=w440:errorcluster, "Save Images.lvclass"=w438:refnum<class "Save Images.lvclass">, "CCDCamera out"=w433:refnum<class "CCDCamera.lvclass">)  [unwired: 7 in]
          n158 = call-dynamic "Get Number of New Images.vi"("error in (no error)"=w440, "Save Images in"=w438) -> ("error out"=w441:errorcluster, "Are the any new img ?"=w443:bool, "Are there any remaining img?"=w442:bool, "Save Images out"=w439:refnum<class "Save Images.lvclass">)  [unwired: 6 in]
          n159 = case shown="False" w443 {
            tunnel: w439 -> [w446 w459]
            tunnel: w441 -> [w445 w450]
            tunnel: [w446 w458] -> w436
            tunnel: [w445 w457] -> w437
            tunnel: w433 -> [w444 w449]
            tunnel: [w444 w448] -> w432
            frame False {
            }
            frame True {
              n160 = call-dynamic "Read Readout Charact.lvclass.vi"("error in (no error)"=w450, "CCDCamera in"=w449) -> ("error out"=w452:errorcluster, "Readout Charact.lvclass"=w455:refnum<class "Readout Charact.lvclass">, "CCDCamera out"=w456:refnum<class "CCDCamera.lvclass">)  [unwired: 7 in]
              n161 = call <vilib>:"High Resolution Relative Seconds.vi"() -> ("relative seconds"=w451:dbl)
              n162 = call-dynamic "Write Third Time.vi"("error in (no error)"=w452, "Third Time"=w451, "Readout Charact in"=w455) -> ("error out"=w453:errorcluster, "Readout Charact out"=w454:refnum<class "Readout Charact.lvclass">)  [unwired: 7 in]
              n163 = call-dynamic "Write Readout Charact.lvclass.vi"("error in (no error)"=w453, "Readout Charact.lvclass"=w454, "CCDCamera in"=w456) -> ("error out"=w447:errorcluster, "CCDCamera out"=w448:refnum<class "CCDCamera.lvclass">)  [unwired: 7 in]
              n164 = call-dynamic "Get Image.vi"("error in (no error)"=w447, "Save Images in"=w459) -> ("error out"=w457:errorcluster, "Save Images out"=w458:refnum<class "Save Images.lvclass">)  [unwired: 8 in]
            }
          }
          n165 = case shown="False" w442 {
            tunnel: w432 -> [w464 w496]
            tunnel: [w468 w497] -> w430
            tunnel: [w467 w498] -> w431
            tunnel: w436 -> [w463 w495]
            tunnel: w437 -> [w462 w494]
            frame False {
              n166 = call-dynamic "Get Image Timings.vi"("error in (no error)"=w462, "Save Images in"=w463) -> ("error out"=w460:errorcluster, "Save Images out"=w461:refnum<class "Save Images.lvclass">)  [unwired: 8 in]
              n167 = call "Write Save Images.lvclass.vi"("error in (no error)"=w460, "Save Images.lvclass"=w461, "CCDCamera in"=w464) -> ("error out"=w466:errorcluster, "CCDCamera out"=w465:refnum<class "CCDCamera.lvclass">)  [unwired: 7 in]
              n168 = call-dynamic "Read Interface.lvclass.vi"("error in (no error)"=w466, "CCDCamera in"=w465) -> ("error out"=w476:errorcluster, "Interface.lvclass"=w475:refnum<class "Interface.lvclass">, "CCDCamera out"=w488:refnum<class "CCDCamera.lvclass">)  [unwired: 7 in]
              n169 = call-dynamic "Read Exposições realizadas.vi"("error in (no error)"=w476, "Interface in"=w475) -> ("error out"=w474:errorcluster, "Exposições realizadas"=w471:dbl, "Interface out"=w473:refnum<class "Interface.lvclass">)  [unwired: 7 in]
              n170 = Increment(x=w471) -> (x+1=w472:dbl)
              n171 = call-dynamic "Write Exposições realizadas.vi"("error in (no error)"=w474, "Exposições realizadas"=w472, "Interface in"=w473) -> ("error out"=w477:errorcluster, "Interface out"=w478:refnum<class "Interface.lvclass">)  [unwired: 7 in]
              n172 = call-dynamic "Read # Images.vi"("error in (no error)"=w477, "Interface in"=w478) -> ("error out"=w480:errorcluster, "# Images"=w483:u32, "Interface out"=w479:refnum<class "Interface.lvclass">)  [unwired: 7 in]
              n173 = Equal?(x=u32 0, y=w483) -> (x = y?=w481:bool)
              n174 = case shown="False" w481 {
                tunnel: [w490 w491] -> w482
                tunnel: w483 -> [w489 w491]
                frame False {
                  n175 = Decrement(x=w489) -> (x-1=w490:u32)
                }
                frame True {
                }
              }
              n176 = call-dynamic "Write # Images.vi"("error in (no error)"=w480, "# Images"=w482, "Interface in"=w479) -> ("error out"=w484:errorcluster, "Interface out"=w485:refnum<class "Interface.lvclass">)  [unwired: 7 in]
              n177 = call "Write Command.vi"("error in (no error)"=w484, "Command"="SAVE IMAGE", "Interface in"=w485) -> ("error out"=w486:errorcluster, "Interface out"=w487:refnum<class "Interface.lvclass">)  [unwired: 7 in]
              n178 = call-dynamic "Write Interface.lvclass.vi"("error in (no error)"=w486, "Interface.lvclass"=w487, "CCDCamera in"=w488) -> ("error out"=w468:errorcluster, "CCDCamera out"=w467:refnum<class "CCDCamera.lvclass">)  [unwired: 7 in]
            }
            frame True {
              n179 = call "Write Save Images.lvclass.vi"("error in (no error)"=w494, "Save Images.lvclass"=w495, "CCDCamera in"=w496) -> ("error out"=w492:errorcluster, "CCDCamera out"=w493:refnum<class "CCDCamera.lvclass">)  [unwired: 7 in]
              n180 = call-dynamic "Read Interface.lvclass.vi"("error in (no error)"=w492, "CCDCamera in"=w493) -> ("error out"=w504:errorcluster, "Interface.lvclass"=w503:refnum<class "Interface.lvclass">, "CCDCamera out"=w501:refnum<class "CCDCamera.lvclass">)  [unwired: 7 in]
              n181 = call "Write Command.vi"("error in (no error)"=w504, "Command"="REPEAT", "Interface in"=w503) -> ("error out"=w499:errorcluster, "Interface out"=w500:refnum<class "Interface.lvclass">)  [unwired: 7 in]
              n182 = call-dynamic "Write Interface.lvclass.vi"("error in (no error)"=w499, "Interface.lvclass"=w500, "CCDCamera in"=w501) -> ("error out"=w497:errorcluster, "CCDCamera out"=w498:refnum<class "CCDCamera.lvclass">)  [unwired: 7 in]
            }
          }
        }
        frame "SAVE IMAGE KINETIC" {
          n183 = flat-sequence {
            tunnel: w524 -> [w582]
            tunnel: w525 -> [w581]
            tunnel: [w580] -> w527
            tunnel: [w579] -> w526
            frame #0 {
              n184 = call-dynamic "Read Readout Charact.lvclass.vi"("error in (no error)"=w582, "CCDCamera in"=w581) -> ("error out"=w574:errorcluster, "Readout Charact.lvclass"=w577:refnum<class "Readout Charact.lvclass">, "CCDCamera out"=w578:refnum<class "CCDCamera.lvclass">)  [unwired: 7 in]
              n185 = call <vilib>:"High Resolution Relative Seconds.vi"() -> ("relative seconds"=w573:dbl)
              n186 = call-dynamic "Write Fourth Time.vi"("error in (no error)"=w574, "Fourth Time"=w573, "Readout Charact in"=w577) -> ("error out"=w575:errorcluster, "Readout Charact out"=w576:refnum<class "Readout Charact.lvclass">)  [unwired: 7 in]
              n187 = call-dynamic "Write Readout Charact.lvclass.vi"("error in (no error)"=w575, "Readout Charact.lvclass"=w576, "CCDCamera in"=w578) -> ("error out"=w579:errorcluster, "CCDCamera out"=w580:refnum<class "CCDCamera.lvclass">)  [unwired: 7 in]
            }
          }
          n188 = call "Read Save Images.lvclass.vi"("error in (no error)"=w526, "CCDCamera in"=w527) -> ("error out"=w534:errorcluster, "Save Images.lvclass"=w535:refnum<class "Save Images.lvclass">, "CCDCamera out"=w533:refnum<class "CCDCamera.lvclass">)  [unwired: 7 in]
          n189 = call-dynamic "Write Image Name.vi"("error in (no error)"=w534, "Save Images in"=w535) -> ("error out"=w541:errorcluster, "Save Images out"=w539:refnum<class "Save Images.lvclass">)  [unwired: 7 in, 1 out]
          n190 = call-dynamic "Save Image.vi"("error in (no error)"=w541, "Save Images in"=w539) -> ("error out"=w540:errorcluster, "Save Images out"=w538:refnum<class "Save Images.lvclass">)  [unwired: 8 in]
          n191 = call-dynamic "Write Image Header.vi"("error in (no error)"=w540, "Save Images in"=w538) -> ("error out"=w537:errorcluster, "Save Images out"=w536:refnum<class "Save Images.lvclass">)  [unwired: 8 in]
          n192 = call-dynamic "Clean Image Graph.vi"("error in (no error)"=w537, "Save Images in"=w536) -> ("error out"=w532:errorcluster, "Save Images out"=w531:refnum<class "Save Images.lvclass">)  [unwired: 8 in]
          n193 = call "Write Last  Image.vi"("error in (no error)"=w532, "Last  Image"=0, "Save Images in"=w531) -> ("error out"=w528:errorcluster, "Save Images out"=w529:refnum<class "Save Images.lvclass">)  [unwired: 7 in]
          n194 = call "Write Save Images.lvclass.vi"("error in (no error)"=w528, "Save Images.lvclass"=w529, "CCDCamera in"=w533) -> ("error out"=w522:errorcluster, "CCDCamera out"=w523:refnum<class "CCDCamera.lvclass">)  [unwired: 7 in]
          n195 = flat-sequence {
            tunnel: w522 -> [w572]
            tunnel: w523 -> [w571]
            tunnel: [w564] -> w515
            tunnel: [w563] -> w516
            frame #0 {
              n196 = call-dynamic "Read Readout Charact.lvclass.vi"("error in (no error)"=w572, "CCDCamera in"=w571) -> ("error out"=w570:errorcluster, "Readout Charact.lvclass"=w569:refnum<class "Readout Charact.lvclass">, "CCDCamera out"=w565:refnum<class "CCDCamera.lvclass">)  [unwired: 7 in]
              n197 = call <vilib>:"High Resolution Relative Seconds.vi"() -> ("relative seconds"=w568:dbl)
              n198 = call-dynamic "Write Fifth Time.vi"("error in (no error)"=w570, "Fifth Time"=w568, "Readout Charact in"=w569) -> ("error out"=w566:errorcluster, "Readout Charact out"=w567:refnum<class "Readout Charact.lvclass">)  [unwired: 7 in]
              n199 = call-dynamic "Write Readout Charact.lvclass.vi"("error in (no error)"=w566, "Readout Charact.lvclass"=w567, "CCDCamera in"=w565) -> ("error out"=w563:errorcluster, "CCDCamera out"=w564:refnum<class "CCDCamera.lvclass">)  [unwired: 7 in]
            }
          }
          n200 = call-dynamic "Read Interface.lvclass.vi"("error in (no error)"=w516, "CCDCamera in"=w515) -> ("error out"=w513:errorcluster, "Interface.lvclass"=w514:refnum<class "Interface.lvclass">, "CCDCamera out"=w509:refnum<class "CCDCamera.lvclass">)  [unwired: 7 in]
          n201 = call-dynamic "Read # Images.vi"("error in (no error)"=w513, "Interface in"=w514) -> ("error out"=w508:errorcluster, "# Images"=w512:u32)  [unwired: 7 in, 1 out]
          n202 = Equal?(x=w512, y=0) -> (x = y?=w510:bool)
          n203 = case shown="True" w510 {
            tunnel: w509 -> [w548 w553]
            tunnel: w508 -> [w547 w552]
            tunnel: [w548 w551] -> w507
            tunnel: [w547 w550] -> w506
            tunnel: [_ w549] -> w505
            frame False {
            }
            frame True {
              n204 = call-dynamic "Read Readout Charact.lvclass.vi"("error in (no error)"=w552, "CCDCamera in"=w553) -> ("error out"=w560:errorcluster, "Readout Charact.lvclass"=w561:refnum<class "Readout Charact.lvclass">, "CCDCamera out"=w562:refnum<class "CCDCamera.lvclass">)  [unwired: 7 in]
              n205 = call "Calculate Delay.vi"("error in (no error)"=w560, "Readout Charact in"=w561) -> ("error out"=w554:errorcluster, "Readout Charact out"=w555:refnum<class "Readout Charact.lvclass">)  [unwired: 8 in]
              n206 = call "Create String Times.vi"("error in (no error)"=w554, "Readout Charact in"=w555) -> ("error out"=w556:errorcluster, "Readout Charact out"=w557:refnum<class "Readout Charact.lvclass">)  [unwired: 8 in]
              n207 = call-dynamic "Read String of the times.vi"("error in (no error)"=w556, "Readout Charact in"=w557) -> ("error out"=w559:errorcluster, "String of the times"=w549:string, "Readout Charact out"=w558:refnum<class "Readout Charact.lvclass">)  [unwired: 7 in]
              n208 = call-dynamic "Write Readout Charact.lvclass.vi"("error in (no error)"=w559, "Readout Charact.lvclass"=w558, "CCDCamera in"=w562) -> ("error out"=w550:errorcluster, "CCDCamera out"=w551:refnum<class "CCDCamera.lvclass">)  [unwired: 7 in]
            }
          }
          n209 = call-dynamic "Read Interface.lvclass.vi"("error in (no error)"=w506, "CCDCamera in"=w507) -> ("error out"=w518:errorcluster, "Interface.lvclass"=w517:refnum<class "Interface.lvclass">, "CCDCamera out"=w521:refnum<class "CCDCamera.lvclass">)  [unwired: 7 in]
          n210 = call-dynamic "Write Timings String.vi"("error in (no error)"=w518, "Timings String"=w505, "Interface in"=w517) -> ("error out"=w519:errorcluster, "Interface out"=w520:refnum<class "Interface.lvclass">)  [unwired: 7 in]
          n211 = call "Write Command.vi"("error in (no error)"=w519, "Command"="IMAGE SAVED", "Interface in"=w520) -> ("error out"=w545:errorcluster, "Interface out"=w544:refnum<class "Interface.lvclass">)  [unwired: 7 in]
          n212 = call-dynamic "Write Interface.lvclass.vi"("error in (no error)"=w545, "Interface.lvclass"=w544, "CCDCamera in"=w521) -> ("error out"=w543:errorcluster, "CCDCamera out"=w542:refnum<class "CCDCamera.lvclass">)  [unwired: 7 in]
        }
        frame "ABORT ACQUISITION" {
          n213 = call "Abort Acquisition.vi"("error in (no error)"=w600, "CCDCamera in"=w599) -> ("error out"=w594:errorcluster, "CCDCamera out"=w593:refnum<class "CCDCamera.lvclass">)  [unwired: 8 in]
          n214 = call-dynamic "Read Interface.lvclass.vi"("error in (no error)"=w594, "CCDCamera in"=w593) -> ("error out"=w591:errorcluster, "Interface.lvclass"=w592:refnum<class "Interface.lvclass">, "CCDCamera out"=w590:refnum<class "CCDCamera.lvclass">)  [unwired: 7 in]
          n215 = call-dynamic "Write # Images.vi"("error in (no error)"=w591, "# Images"=u32 0, "Interface in"=w592) -> ("error out"=w598:errorcluster, "Interface out"=w595:refnum<class "Interface.lvclass">)  [unwired: 7 in]
          n216 = call-dynamic "Write Abort.vi"("error in (no error)"=w598, "Abort"=FALSE, "Interface in"=w595) -> ("error out"=w587:errorcluster, "Interface out"=w586:refnum<class "Interface.lvclass">)  [unwired: 7 in]
          n217 = call "Write Command.vi"("error in (no error)"=w587, "Command"="ACQUISITION ABORTED", "Interface in"=w586) -> ("error out"=w583:errorcluster, "Interface out"=w584:refnum<class "Interface.lvclass">)  [unwired: 7 in]
          n218 = call-dynamic "Write Interface.lvclass.vi"("error in (no error)"=w583, "Interface.lvclass"=w584, "CCDCamera in"=w590) -> ("error out"=w589:errorcluster, "CCDCamera out"=w588:refnum<class "CCDCamera.lvclass">)  [unwired: 7 in]
        }
        frame "STOP ACQUISITION" {
          n219 = call-dynamic "Read Interface.lvclass.vi"("error in (no error)"=w611, "CCDCamera in"=w612) -> ("error out"=w609:errorcluster, "Interface.lvclass"=w610:refnum<class "Interface.lvclass">, "CCDCamera out"=w608:refnum<class "CCDCamera.lvclass">)  [unwired: 7 in]
          n220 = call-dynamic "Write # Images.vi"("error in (no error)"=w609, "# Images"=u32 0, "Interface in"=w610) -> ("error out"=w616:errorcluster, "Interface out"=w615:refnum<class "Interface.lvclass">)  [unwired: 7 in]
          n221 = call-dynamic "Write Stop Acq.vi"("error in (no error)"=w616, "Stop Acq"=FALSE, "Interface in"=w615) -> ("error out"=w602:errorcluster, "Interface out"=w605:refnum<class "Interface.lvclass">)  [unwired: 7 in]
          n222 = call "Write Command.vi"("error in (no error)"=w602, "Command"="ACQUISITION STOPED", "Interface in"=w605) -> ("error out"=w603:errorcluster, "Interface out"=w604:refnum<class "Interface.lvclass">)  [unwired: 7 in]
          n223 = call-dynamic "Write Interface.lvclass.vi"("error in (no error)"=w603, "Interface.lvclass"=w604, "CCDCamera in"=w608) -> ("error out"=w606:errorcluster, "CCDCamera out"=w607:refnum<class "CCDCamera.lvclass">)  [unwired: 7 in]
        }
        frame "N/A" {
        }
        frame "SET TEMPERATURE" {
          n224 = call "Write Temperature to Cooler.vi"("error in (no error)"=w629, "CCDCamera in"=w630) -> ("error out"=w620:errorcluster, "CCDCamera out"=w619:refnum<class "CCDCamera.lvclass">)  [unwired: 8 in]
          n225 = call-dynamic "Read Cooler.lvclass.vi"("error in (no error)"=w620, "CCDCamera in"=w619) -> ("error out"=w622:errorcluster, "Cooler.lvclass"=w621:refnum<class "Cooler.lvclass">, "CCDCamera out"=w623:refnum<class "CCDCamera.lvclass">)  [unwired: 7 in]
          n226 = call "Verify Cooler.vi"("error in (no error)"=w622, "Cooler in"=w621) -> ("error out"=w626:errorcluster, "coolerStatus"=w628:bool, "Cooler out"=w627:refnum<class "Cooler.lvclass">)  [unwired: 7 in]
          n227 = case shown="True" w628 {
            tunnel: w627 -> [w634 w638]
            tunnel: [w634 w637] -> w625
            tunnel: w626 -> [w633 w636]
            tunnel: [w633 w635] -> w624
            frame False {
            }
            frame True {
              n228 = call "Set Temperature.vi"("error in (no error)"=w636, "Cooler in"=w638) -> ("error out"=w635:errorcluster, "Cooler out"=w637:refnum<class "Cooler.lvclass">)  [unwired: 8 in]
            }
          }
          n229 = call-dynamic "Write Cooler.lvclass.vi"("error in (no error)"=w624, "Cooler.lvclass"=w625, "CCDCamera in"=w623) -> ("error out"=w632:errorcluster, "CCDCamera out"=w631:refnum<class "CCDCamera.lvclass">)  [unwired: 7 in]
        }
        frame "TURN COOLER ON" {
          n230 = call-dynamic "Read Cooler.lvclass.vi"("error in (no error)"=w641, "CCDCamera in"=w642) -> ("error out"=w646:errorcluster, "Cooler.lvclass"=w643:refnum<class "Cooler.lvclass">, "CCDCamera out"=w647:refnum<class "CCDCamera.lvclass">)  [unwired: 7 in]
          n231 = call "Cooler ON.vi"("error in (no error)"=w646, "Cooler in"=w643) -> ("error out"=w645:errorcluster, "Cooler out"=w644:refnum<class "Cooler.lvclass">)  [unwired: 8 in]
          n232 = call-dynamic "Write Cooler.lvclass.vi"("error in (no error)"=w645, "Cooler.lvclass"=w644, "CCDCamera in"=w647) -> ("error out"=w640:errorcluster, "CCDCamera out"=w639:refnum<class "CCDCamera.lvclass">)  [unwired: 7 in]
        }
        frame "TURN COOLER OFF" {
          n233 = call-dynamic "Read Cooler.lvclass.vi"("error in (no error)"=w654, "CCDCamera in"=w655) -> ("error out"=w648:errorcluster, "Cooler.lvclass"=w651:refnum<class "Cooler.lvclass">, "CCDCamera out"=w656:refnum<class "CCDCamera.lvclass">)  [unwired: 7 in]
          n234 = call "Cooler OFF.vi"("error in (no error)"=w648, "Cooler in"=w651) -> ("error out"=w649:errorcluster, "Cooler out"=w650:refnum<class "Cooler.lvclass">)  [unwired: 8 in]
          n235 = call-dynamic "Write Cooler.lvclass.vi"("error in (no error)"=w649, "Cooler.lvclass"=w650, "CCDCamera in"=w656) -> ("error out"=w652:errorcluster, "CCDCamera out"=w653:refnum<class "CCDCamera.lvclass">)  [unwired: 7 in]
        }
      }
      n236 = call-dynamic "Read Interface.lvclass.vi"("error in (no error)"=w231, "CCDCamera in"=w230) -> ("error out"=w223:errorcluster, "Interface.lvclass"=w203:refnum<class "Interface.lvclass">, "CCDCamera out"=w224:refnum<class "CCDCamera.lvclass">)  [unwired: 7 in]
      n237 = call "Write Current CCD Class.vi"("error in (no error)"=w223, "CCD Class"=w224, "Channel Manager in"=w222) -> ("error out"=w221:errorcluster, "Channel Manager out"=w220:refnum<class "Channel Manager.lvclass">)  [unwired: 7 in]
      n238 = call "Return Current RxTx.vi"("error in (no error)"=w221, "Channel Manager in"=w220) -> ("error out"=w213:errorcluster, "RxTx"=w214:refnum<class "RxTx.lvclass">, "Channel Manager out"=w210:refnum<class "Channel Manager.lvclass">)  [unwired: 7 in]
      n239 = call-dynamic "Write Interface.lvclass.vi"("error in (no error)"=w213, "Interface.lvclass"=w203, "RxTx in"=w214) -> ("error out"=w215:errorcluster, "RxTx out"=w216:refnum<class "RxTx.lvclass">)  [unwired: 7 in]
      n240 = call "Verify Command.vi"("error in (no error)"=w215, "RxTx in"=w216) -> ("error out"=w218:errorcluster, "Empyt string?"=w217:bool, "RxTx out"=w219:refnum<class "RxTx.lvclass">)  [unwired: 7 in]
      n241 = case shown="False" w217 {
        tunnel: w218 -> [w246 w247]
        tunnel: w219 -> [w245 w248]
        tunnel: [w244 w248] -> w212
        tunnel: [w243 w247] -> w211
        frame False {
          n242 = call "Enqeue B Message.vi"("error in (no error)"=w246, "RxTx in"=w245) -> ("error out"=w243:errorcluster, "RxTx out"=w244:refnum<class "RxTx.lvclass">)  [unwired: 8 in]
        }
        frame True {
        }
      }
      n243 = call "Write Current RxTx.vi"("error in (no error)"=w211, "RxTx"=w212, "Channel Manager in"=w210) -> ("error out"=w191:errorcluster, "Channel Manager out"=w192:refnum<class "Channel Manager.lvclass">)  [unwired: 7 in]
    }
    n244 = Boolean To (0,1)(Boolean=w185) -> (0, 1=w184:i16[])
    n245 = Add Array Elements(numeric array=w184) -> (sum=w183:i16)
    n246 = Greater Or Equal?(x=w183, y=1) -> (x >= y?=w181:bool)
    n247 = Wait Until Next ms Multiple(millisecond multiple=u32 5) -> ()  [unwired: 1 out]
  }
  n248 = call-dynamic "Read Available Cameras.vi"("error in (no error)"=w5, "Channel Manager in"=w4) -> ("error out"=w1:errorcluster, "Available Cameras"=w3:u8, "Channel Manager out"=w2:refnum<class "Channel Manager.lvclass">)  [unwired: 7 in]
  n249 = for {
    N: w3 -> [_]
    shift-right: [w662] -> _
    shift-left: w2 -> [w659]
    shift-right: [w663] -> _
    shift-left: w1 -> [w658]
    i -> [w657]
    n250 = call-dynamic "Write Current Camera.vi"("error in (no error)"=w658, "Current Camera"=w657, "Channel Manager in"=w659) -> ("error out"=w661:errorcluster, "Channel Manager out"=w660:refnum<class "Channel Manager.lvclass">)  [unwired: 7 in]
    n251 = call "Set Current CCD.vi"("error in (no error)"=w661, "Channel Manager in"=w660) -> ("error out"=w682:errorcluster, "Channel Manager out"=w683:refnum<class "Channel Manager.lvclass">)  [unwired: 8 in]
    n252 = call "Return Current CCD Class.vi"("error in (no error)"=w682, "Channel Manager in"=w683) -> ("error out"=w666:errorcluster, "CCD Class"=w667:refnum<class "CCDCamera.lvclass">, "Channel Manager out"=w681:refnum<class "Channel Manager.lvclass">)  [unwired: 7 in]
    n253 = call-dynamic "Read Cooler.lvclass.vi"("error in (no error)"=w666, "CCDCamera in"=w667) -> ("error out"=w677:errorcluster, "Cooler.lvclass"=w676:refnum<class "Cooler.lvclass">, "CCDCamera out"=w680:refnum<class "CCDCamera.lvclass">)  [unwired: 7 in]
    n254 = call-dynamic "Write Temperature.vi"("error in (no error)"=w677, "Temperature"=20.0, "Cooler in"=w676) -> ("error out"=w679:errorcluster, "Cooler out"=w678:refnum<class "Cooler.lvclass">)  [unwired: 7 in]
    n255 = call "Verify Cooler.vi"("error in (no error)"=w679, "Cooler in"=w678) -> ("error out"=w673:errorcluster, "coolerStatus"=w671:bool, "Cooler out"=w672:refnum<class "Cooler.lvclass">)  [unwired: 7 in]
    n256 = case shown="True" w671 {
      tunnel: w672 -> [w685 w689]
      tunnel: [w685 w688] -> w674
      tunnel: w673 -> [w684 w687]
      tunnel: [w684 w686] -> w675
      frame False {
      }
      frame True {
        n257 = call "Set Temperature.vi"("error in (no error)"=w687, "Cooler in"=w689) -> ("error out"=w686:errorcluster, "Cooler out"=w688:refnum<class "Cooler.lvclass">)  [unwired: 8 in]
      }
    }
    n258 = call-dynamic "Write Cooler.lvclass.vi"("error in (no error)"=w675, "Cooler.lvclass"=w674, "CCDCamera in"=w680) -> ("error out"=w670:errorcluster, "CCDCamera out"=w669:refnum<class "CCDCamera.lvclass">)  [unwired: 7 in]
    n259 = call "Shutdown Camera.vi"("error in (no error)"=w670, "CCDCamera in"=w669) -> ("error out"=w664:errorcluster, "CCDCamera out"=w665:refnum<class "CCDCamera.lvclass">)  [unwired: 8 in]
    n260 = call "Write Current CCD Class.vi"("error in (no error)"=w664, "CCD Class"=w665, "Channel Manager in"=w681) -> ("error out"=w663:errorcluster, "Channel Manager out"=w662:refnum<class "Channel Manager.lvclass">)  [unwired: 7 in]
  }
